vi "Read Profiles(for High-Speed Data Communication).vi"(0 "Device ID (0)":i32, 5 "Timeout":u32, 11 "error in (no error)":errorcluster {"code" format="%.0x"}) -> (3 "Profile Info":T1, 4 "Device ID out":i32, 6 "Profile Data":u32[](array[numeric]), 8 "Rsp Profile Cnt":u32, 10 "Notify":u32, 14 "Buf Usage Rate":u32, 15 "error out":errorcluster {"code" format="%.0x"})   [LabVIEW 2010, in "KEYENCE LJ-X8000A.lvlib"]
doc: "Profile data will be acquired by high-speed communication.\nProfile data will be stored in a unit of 0.01 ƒÊm.\n\n<B>Note</B>:\nRefer to the reference manual for contents (storage order and size) of data to be stored in profile data."
uses:
  KEYENCE LJ-X8000A.lvlib
  Clusters/Profile Info.ctl
panel:
  # "(c) 2019 KEYENCE CORPORATION.  ALL RIGHTS RESERVED."
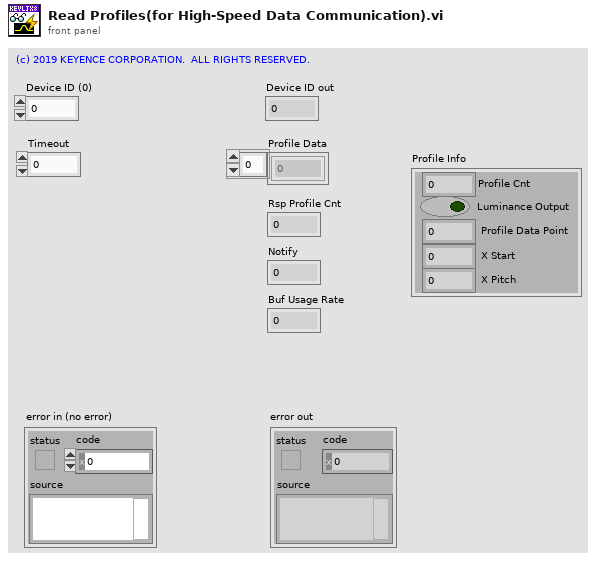
[diagram p1: front panel]
types:
  T1 = typedef "KEYENCE LJ-X8000A.lvlib/Profile Info.ctl" = cluster{"Profile Cnt":u8, "Luminance Output":bool, " Profile Data Point":u16, " X Start":i32, " X Pitch":i32}
  T2 = cluster{"byProfileCount":u8, "reserve":u8, "byLuminanceOutput":u8, "reserve":u8, "wProfileDataCount":u16, "reserve":u8, "reserve":u8, "lXStart":i32, "lXPitch":i32}
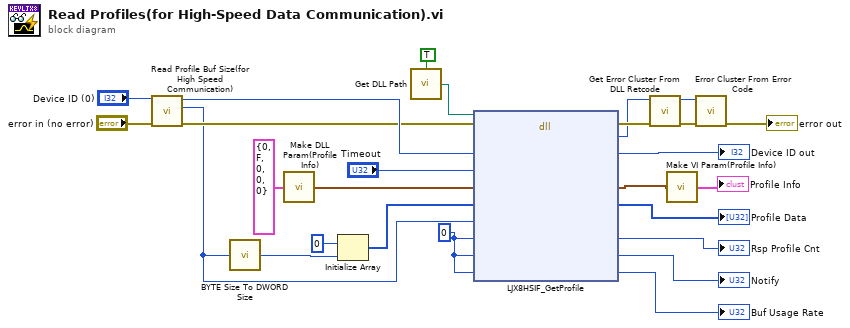
[diagram p0: block diagram]
diagram:
  w14 = u32 0 ("pdwRspProfileCnt")
  n1 = call "Read Profile Buf Size(for High Speed Communication).vi"("error in (no error)"="error in (no error)", "Device ID (0)"="Device ID (0)") -> ("error out"=w18:errorcluster, "Profile Buf Size"=w7:u32, "Device ID out"=w20:i32)  [unwired: 7 in]
  n2 = call "BYTE Size To DWORD Size.vi"("BYTE Size"=w7) -> ("DWORD Size"=w8:u32)
  n3 = call "Make DLL Param(Profile Info).vi"("Profile Info"=T1 {"Profile Cnt"=0, "Luminance Output"=FALSE, " Profile Data Point"=0, " X Start"=0, " X Pitch"=0}) -> ("DLL Parameter"=w5:T2)
  n4 = Initialize Array(u32 0, w8) -> (w16:u32[])
  n5 = call "Get DLL Path.vi"("isWrapperDLL (False)"=TRUE) -> ("DLL Path"=w12:path)  [unwired: 2 in]
  n6 = dll-call lib="C:/Program Files (x86)/National Instruments/LabVIEW 2018/instr.lib/KEYENCE LJ-X8000/LJX8_HighSpeedWrapper.*" fn="LJX8HSIF_GetProfile"(path in=w12, error in=w18, "lDeviceId"=w20, "dwTimeout"="Timeout", "pProfileInfo"=w5, "pdwData"=w16, "dwDataSize"=w7, "pdwRspProfileCnt"=w14, "pdwNotify"=w14, "pdwUsageRate"=w14) -> (error out=w11:errorcluster, "lRetCode"=w9:i32, "lDeviceId"=→"Device ID out":i32, "pProfileInfo"=w4:T2, "pdwData"=→"Profile Data":u32[], "pdwRspProfileCnt"=→"Rsp Profile Cnt":u32, "pdwNotify"=→"Notify":u32, "pdwUsageRate"=→"Buf Usage Rate":u32)  [unwired: 3 in, 1 out]
  n7 = call "Get Error Cluster From DLL Retcode.vi"("error in (no error)"=w11, "DLL Return Code"=w9) -> ("error out"=w10:errorcluster, "VI Error Code"=w1:i32)  [unwired: 8 in]
  n8 = call "Make VI Param(Profile Info).vi"("pProfileInfo"=w4) -> ("Profile Info"=→"Profile Info":T1)
  n9 = call <vilib>:"Error Cluster From Error Code.vi"("error in (no error)"=w10, "error code (0)"=w1) -> ("error out"=→"error out":errorcluster)  [unwired: 7 in]
